vi "Write to RT Error Log.vi"(8 "error in (no error)":errorcluster, 11 "Log Entry":string) -> (0 "error out":errorcluster)   [LabVIEW 2013]
uses:
  Globals/Global - Configuration Options.vi
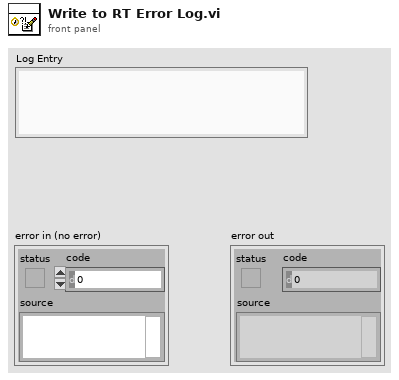
[diagram p1: front panel]
types:
  T1 = enum16{"open", "replace", "create", "open or create", "replace or create", "replace or create with confirmation"}
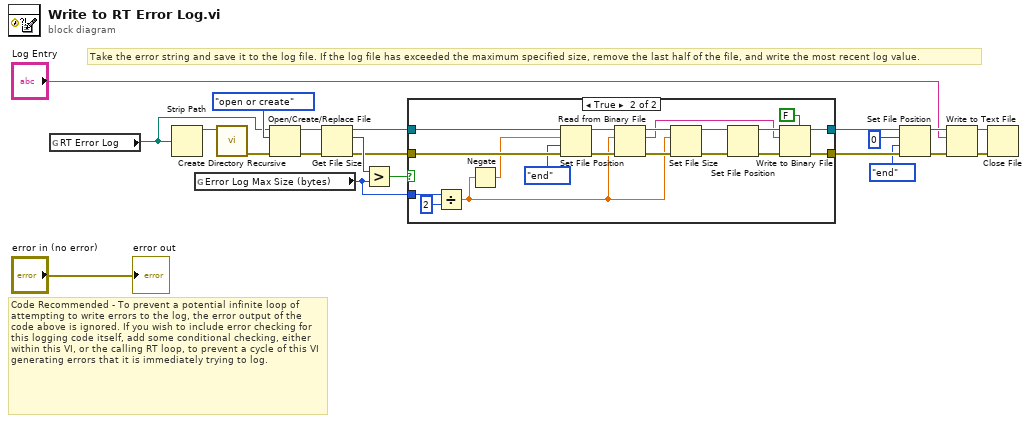
[diagram p0: block diagram]
diagram:
  # "Code Recommended - To prevent a potential infinite loop of attempting to write errors to the log, the error output of the code above is ignored. If you wish to include error checking for this logging code itself, add some conditional checking, either within this VI, or the calling RT loop, to prevent a cycle of this VI generating errors that it is immediately trying to log."
  # "Take the error string and save it to the log file. If the log file has exceeded the maximum specified size, remove the last half of the file, and write the most recent log value."
  n1 = global read "Global - Configuration Options.vi" "RT Error Log"() -> (w4:path)
  n2 = Strip Path(path=w4) -> (stripped path=w5:path)  [unwired: 1 out]
  n3 = global read "Global - Configuration Options.vi" "Error Log Max Size (bytes)"() -> (w7:i64)
  n4 = call <vilib>:"Create Directory Recursive.vi"("directory"=w5) -> ("error out"=w6:errorcluster)  [unwired: 4 in, 2 out]
  n5 = Open/Create/Replace File(file path (use dialog)=w4, error in=w6, operation (0:open)=T1."open or create") -> (refnum out=w8:refnum<file>, error out=w9:errorcluster)  [unwired: 2 in, 2 out]
  n6 = Get File Size(file=w8, error in=w9) -> (refnum out=w14:refnum<file>, size (in bytes)=w16:i64, 0:w13:errorcluster)
  n7 = Greater?(x=w16, y=w7) -> (0:w15:bool)
  n8 = case shown="True" w15 {
    tunnel: w14 -> [w23 w41]
    tunnel: w13 -> [w22 w42]
    tunnel: w7 -> [_ w38]
    tunnel: [w23 w26] -> w12
    tunnel: [w22 w25] -> w11
    frame False {
    }
    frame True {
      n9 = Divide(x=w38, y=i64 2) -> (x/y=w33:dbl)
      n10 = Negate(x=w33) -> (-x=w24:dbl)
      n11 = Set File Position(offset (in bytes) (0)=w24, refnum=w41, from (0:start)=enum16{"start", "end", "current"}."end", error in=w42) -> (refnum out=w36:refnum<file>, error out=w37:errorcluster)
      n12 = Read from Binary File(8:w37, 10:w33, 11:w36) -> (0:w34:errorcluster, 2:w27:string, 3:w35:refnum<file>)  [unwired: 3 in, 1 out]
      n13 = Set File Size(4:w34, 6:w33, 7:w35) -> (0:w32:errorcluster, 3:w31:refnum<file>)
      n14 = Set File Position(refnum=w31, error in=w32) -> (refnum out=w29:refnum<file>, error out=w30:errorcluster)  [unwired: 2 in]
      n15 = Write to Binary File(file (use dialog)=w29, data=w27, error in=w30, 5:FALSE ("prepend array or string size? (T)")) -> (refnum out=w26:refnum<file>, error out=w25:errorcluster)  [unwired: 2 in, 1 out]
    }
  }
  n16 = Set File Position(offset (in bytes) (0)=i64 0, refnum=w12, from (0:start)=enum16{"start", "end", "current"}."end", error in=w11) -> (refnum out=w19:refnum<file>, error out=w18:errorcluster)
  n17 = Write to Text File(file (use dialog)=w19, text="Log Entry", error in=w18) -> (refnum out=w21:refnum<file>, error out=w20:errorcluster)  [unwired: 1 in, 1 out]
  n18 = Close File(refnum=w21, error in=w20) -> ()  [unwired: 2 out]
  "error out" <- "error in (no error)"
